vi "获取质心方式.vi"(0 "Image":T2, 1 "中心点":u16(ring) items=["自动", "自动获取质心", "手动取心"], 2 "X Centroid":sgl, 3 "Y Centroid":sgl, 4 "ROI":T1, 5 "error in (no error)":errorcluster, 6 "是否加中心线":bool, 7 "第一点x值，y=0":sgl, 9 "第二点x值,y=479":dbl, 11 "第一点y值，x=0":sgl, 12 "是否加椭圆线":bool, 13 "第二点y值，x=639":sgl) -> (10 "是否手动取点":bool, 14 "Image Out 2":T2, 15 "质心坐标X":dbl, 16 "质心坐标Y":dbl, 17 "手动取点x":i32, 18 "手动取点y":i32, 19 "error out":errorcluster)   [LabVIEW 2015]
uses:
  <vilib>/vision/Image Controls.llb/IMAQ Image.ctl
  <vilib>/vision/NI_Vision_Development_Module.lvlib
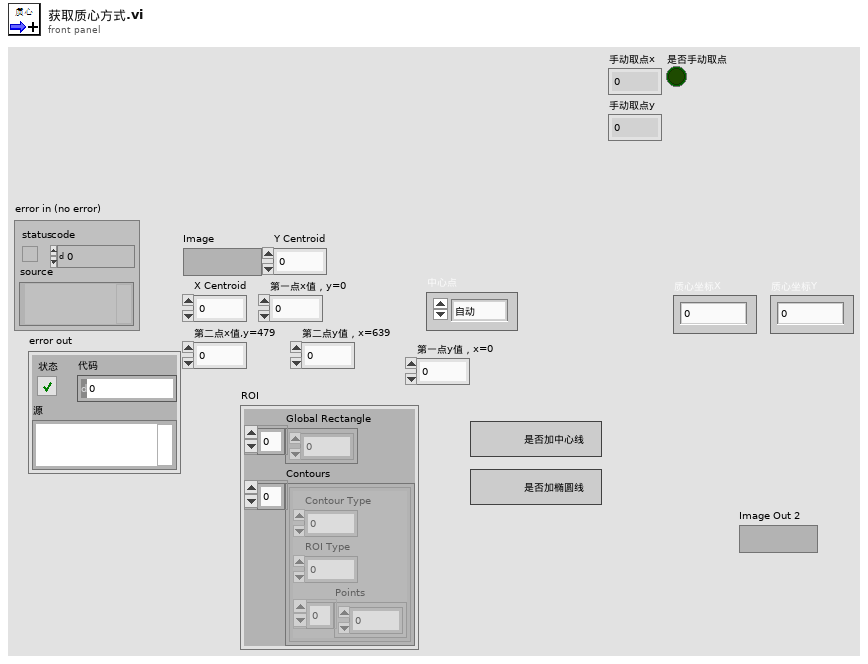
[diagram p1: front panel]
types:
  T1 = cluster{"Global Rectangle":i32[], "Contours":cluster{"Contour Type":u32, "ROI Type":u32, "Points":i32[]}[]}
  T2 = typedef "IMAQ Image.ctl" = refnum<image>
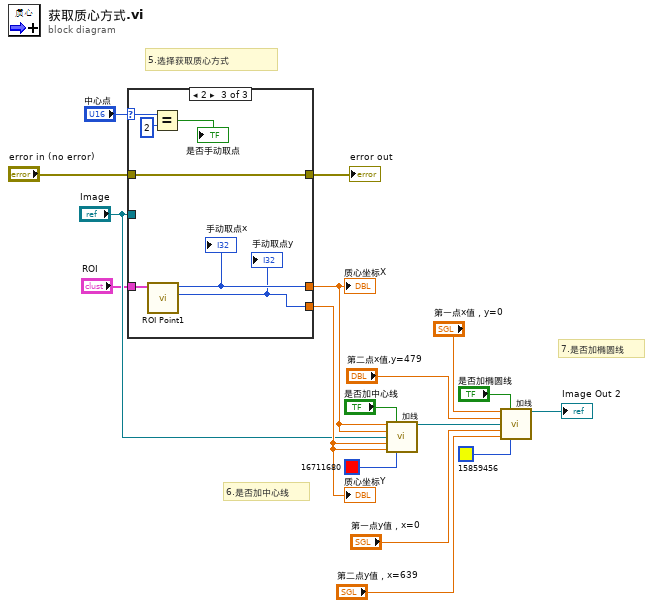
[diagram p0: block diagram]
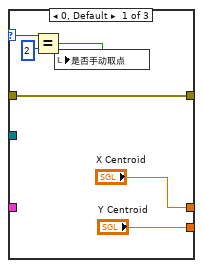
[diagram p2: hidden frame]
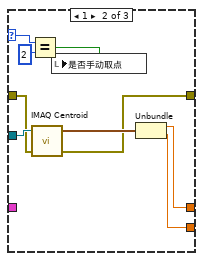
[diagram p3: hidden frame]
diagram:
  # "7.是否加椭圆线"
  # "6.是否加中心线"
  # "5.选择获取质心方式"
  n1 = case shown="2" "中心点" {
    selector: "中心点" -> [w19 w24 w35]
    tunnel: ["Y Centroid" w29 w37] -> w17
    tunnel: ["X Centroid" w30 w38] -> w16
    tunnel: "Image" -> [_ w32 _]
    tunnel: [w21 w28 w39] -> w2
    tunnel: "error in (no error)" -> [w21 w27 w39]
    tunnel: "ROI" -> [_ _ w36]
    frame 0, Default {
      n2 = Equal?(x=w19, y=u16 2) -> (x = y?=w18:bool)
      n3 = local write "是否手动取点"(w18) -> ()
    }
    frame 1 {
      n4 = Equal?(x=w24, y=u16 2) -> (x = y?=w25:bool)
      n5 = call "IMAQ Centroid"("error in (no error)"=w27, "Image"=w32) -> ("error out"=w28:errorcluster, "Centroid"=w31:cluster{"X Centroid":sgl, "Y Centroid":sgl})  [unwired: 1 in, 1 out]
      n6 = local write "是否手动取点"(w25) -> ()
      n7 = Unbundle(w31) -> ("X Centroid"=w30:sgl, "Y Centroid"=w29:sgl)
    }
    frame 2 {
      n8 = call "ROI Point1.vi"("ROI"=w36) -> ("y"=w37:i32, "x"=w38:i32)  [unwired: 9 in]
      "手动取点x" <- w38
      "手动取点y" <- w37
      n9 = Equal?(x=w35, y=u16 2) -> (x = y?=→"是否手动取点":bool)
    }
  }
  "质心坐标X" <- w16
  "质心坐标Y" <- w17
  "error out" <- w2
  n10 = call "加线.vi"("质心X"=w16, "是否加线"="是否加中心线", "质心X 2"=w16, "Image in"="Image", "质心Y"=w17, "质心Y 2"=w17, "Color"=u32 16711680) -> ("Image Out 2"=w14:T2)  [unwired: 8 in]
  n11 = call "加线.vi"("质心X"="第一点x值，y=0", "是否加线"="是否加椭圆线", "质心X 2"="第二点x值,y=479", "Image in"=w14, "质心Y"="第一点y值，x=0", "质心Y 2"="第二点y值，x=639", "Color"=u32 15859456) -> ("Image Out 2"=→"Image Out 2":T2)  [unwired: 8 in]
